vi "Legendre Polynomial_Semi Normalized (1D).vi"(8 "m":i32, 9 "n":i32, 11 "X":dbl[](array[numeric])) -> (3 "Snm(X)":dbl[](array[numeric]))   [LabVIEW 2017, in "NI_AAL_Polynomial.lvlib"]
uses:
  <vilib>/Analysis/NI_AAL_Polynomial.lvlib
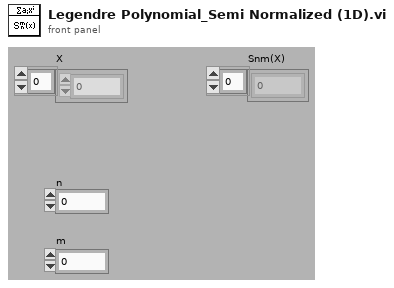
[diagram p1: front panel]
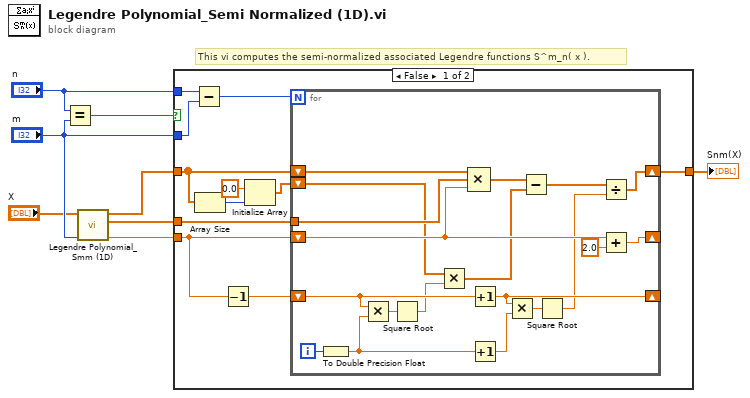
[diagram p0: block diagram]
diagram:
  # "This vi computes the semi-normalized associated Legendre functions S^m_n( x )."
  n1 = Equal?(x="n", y="m") -> (x = y?=w8:bool)
  n2 = call <vilib>:"Legendre Polynomial_Smm (1D).vi"("m"="m", "X In"="X") -> ("2m+1"=w5:dbl, "X Out"=w4:dbl[], "Smm(X)"=w6:dbl[])  [unwired: 7 out]
  n3 = case shown="False" w8 {
    tunnel: w6 -> [w10 w39]
    tunnel: w5 -> [w15 _]
    tunnel: w4 -> [w16 _]
    tunnel: "n" -> [w19 _]
    tunnel: [w13 w39] -> w1
    tunnel: "m" -> [w18 _]
    frame False {
      n4 = Subtract(x=w19, y=w18) -> (x-y=w17:i32)
      n5 = Array Size(array=w10) -> (size(s)=w12:i32)
      n6 = Decrement(x=w15) -> (x-1=w14:dbl)
      n7 = Initialize Array(0.0 ("S^m_m"), w12) -> (w9:dbl[])
      n8 = for {
        N: w17 -> [_]
        shift-right: [w22] -> w13
        shift-left: w10 -> [w37]
        shift-left: w9 -> [w29]
        tunnel: w16 -> [w38]
        shift-right: [w35] -> _
        shift-left: w15 -> [w36]
        shift-right: [w24] -> _
        shift-left: w14 -> [w32]
        i -> [w33]
        n9 = To Double Precision Float(number=w33) -> (double precision float=w26:dbl)
        n10 = Multiply(x=w32, y=w26) -> (x*y=w31:dbl)
        n11 = Square Root(x=w31) -> (sqrt(x)=w30:dbl)
        n12 = Multiply(x=w29, y=w30) -> (x*y=w27:dbl[])
        n13 = Compound Arithmetic op=MULTIPLY(w37, w38, w36) -> (w28:dbl[])
        n14 = Increment(x=w32) -> (x+1=w24:dbl)
        n15 = Increment(x=w26) -> (x+1=w23:dbl)
        n16 = Multiply(x=w24, y=w23) -> (x*y=w25:dbl)
        n17 = Subtract(x=w28, y=w27) -> (x-y=w21:dbl[])
        n18 = Square Root(x=w25) -> (sqrt(x)=w20:dbl)
        n19 = Divide(x=w21, y=w20) -> (x/y=w22:dbl[])
        n20 = Add(x=w36, y=2.0) -> (x+y=w35:dbl)
      }
    }
    frame True {
    }
  }
  "Snm(X)" <- w1
